vi "visitRectangle.vi"(8 "error in (no error)":errorcluster, 10 "Rectangle":refnum<class "Rectangle.lvclass">, 11 "XMLExportVisitor in":refnum<class "XMLExportVisitor.lvclass">) -> (0 "error out":errorcluster, 2 "xml string":string, 3 "XMLExportVisitor out":refnum<class "XMLExportVisitor.lvclass">)   [LabVIEW 2017, in "XMLExportVisitor.lvclass"]
uses:
  XMLExportVisitor.lvclass
  Rectangle Class/Rectangle.lvclass
  Rectangle Class/Rectangle.lvclass/Rectangle.ctl
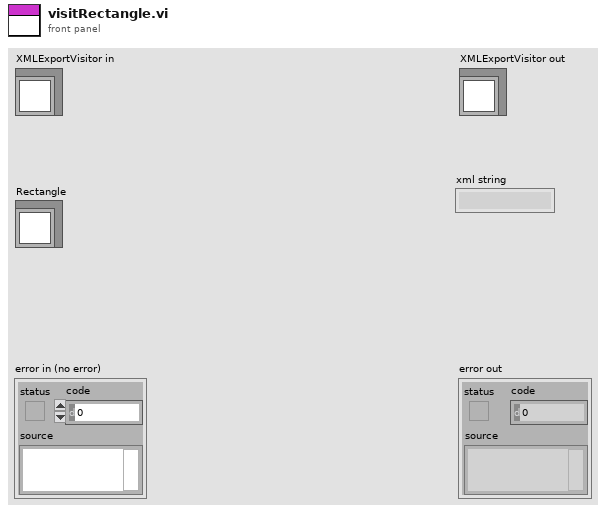
[diagram p1: front panel]
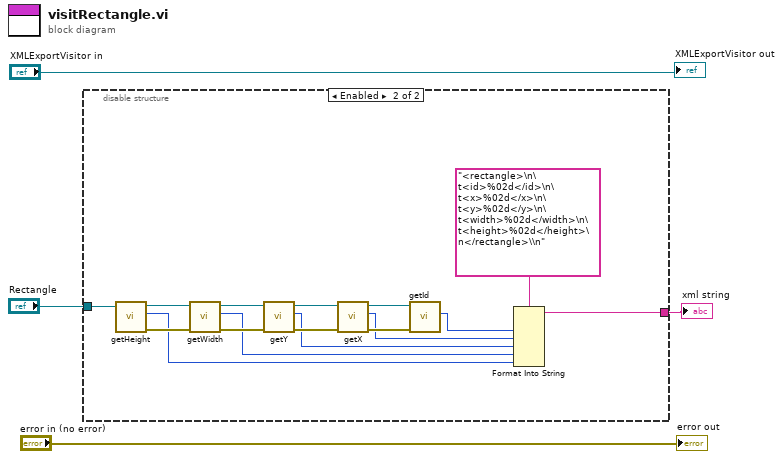
[diagram p0: block diagram]
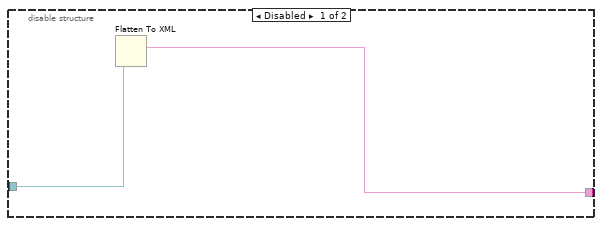
[diagram p2: hidden frame]
diagram:
  n1 = disable-structure shown="Enabled" {
    disable-tunnel: "Rectangle" -> [w6 w22]
    disable-tunnel: [w5 w15] -> w1
    frame Disabled {
      n2 = Flatten To XML(anything=w6) -> (xml string=w5:string)
    }
    frame Enabled {
      n3 = call "getHeight.vi"("Rectangle in"=w22) -> ("error out"=w20:errorcluster, "height"=w7:i32, "Rectangle out"=w21:refnum<class "Rectangle.lvclass">)  [unwired: 8 in]
      n4 = call "getWidth.vi"("error in (no error)"=w20, "Rectangle in"=w21) -> ("error out"=w18:errorcluster, "width"=w8:i32, "Rectangle out"=w19:refnum<class "Rectangle.lvclass">)  [unwired: 7 in]
      n5 = call "getY.vi"("error in (no error)"=w18, "Rectangle in"=w19) -> ("error out"=w16:errorcluster, "y"=w9:i32, "Rectangle out"=w17:refnum<class "Rectangle.lvclass">)  [unwired: 7 in]
      n6 = call "getX.vi"("error in (no error)"=w16, "Rectangle in"=w17) -> ("error out"=w12:errorcluster, "x"=w10:i32, "Rectangle out"=w13:refnum<class "Rectangle.lvclass">)  [unwired: 7 in]
      n7 = call "getId.vi"("error in (no error)"=w12, "Rectangle in"=w13) -> ("id"=w11:i32)  [unwired: 7 in, 2 out]
      n8 = Format Into String(format string="<rectangle>\n\t<id>%02d</id>\n\t<x>%02d</x>\n\t<y>%02d</y>\n\t<width>%02d</width>\n\t<height>%02d</height>\n</rectangle>\\n", w11, w10, w9, w8, w7) -> (resulting string=w15:string)  [unwired: 2 in, 1 out]
    }
  }
  "xml string" <- w1
  "error out" <- "error in (no error)"
  "XMLExportVisitor out" <- "XMLExportVisitor in"
